vi "Update Module Execution Status.vi"(8 "error in (no error)":errorcluster, 10 "Running?":bool) -> (0 "error out":errorcluster)   [LabVIEW 2019, in "Display.lvlib"]
doc: "Broadcast event to specify whether or not the module is running.\n_____\nBased on Delacor QMH Project Template 4.2.1.64."
uses:
  Display.lvlib
  Get Module Execution Status Argument--cluster.ctl
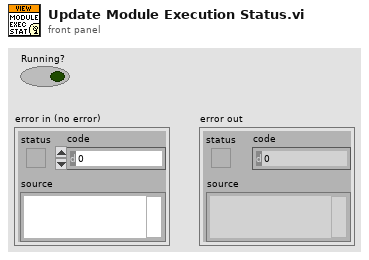
[diagram p1: front panel]
types:
  T1 = typedef "Display.lvlib/Get Module Execution Status Argument--cluster.ctl" = cluster{"Running?":bool}
  T2 = typedef "Display.lvlib/Broadcast Events--cluster.ctl" = cluster{"Module Did Init":refnum<user-event>, "Status Updated":refnum<user-event>, "Error Reported":refnum<user-event>, "Module Did Stop":refnum<user-event>, "Update Module Execution Status":refnum<user-event>}
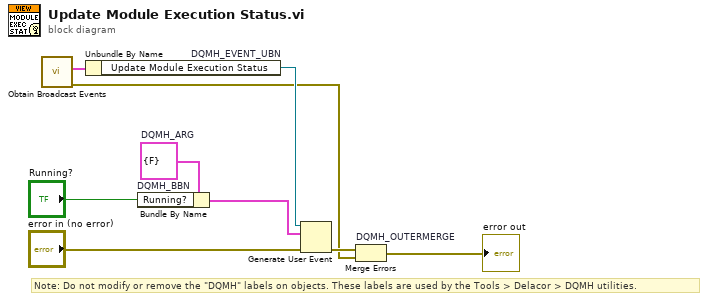
[diagram p0: block diagram]
diagram:
  w4 = T1 {"Running?"=FALSE}  # DQMH_ARG
  # "Note: Do not modify or remove the \"DQMH\" labels on objects. These labels are used by the Tools > Delacor > DQMH utilities."
  n1 = call "Obtain Broadcast Events.vi"() -> ("error out"=w2:errorcluster, "Display Broadcast Events"=w1:T2)  [unwired: 10 in]
  n2 = Unbundle By Name "DQMH_EVENT_UBN"(w1) -> ("Update Module Execution Status"=w5:refnum<user-event>)
  n3 = Bundle By Name "DQMH_BBN"(cluster=w4, "Running?"="Running?") -> (w6:T1)
  n4 = Generate User Event(user event=w5, event data cluster=w6, error in="error in (no error)") -> (error out=w7:errorcluster)  [unwired: 1 in, 1 out]
  n5 = Merge Errors "DQMH_OUTERMERGE"(w7, w2) -> (→"error out":errorcluster)
